vi "ProdaNG.CreateProductComponent.vi"(4 "component serialNo":string, 6 "component wabcoNo":string, 8 "error in (no error)":errorcluster, 9 "product serialNo":string, 10 "product wabcoNo":string, 11 "dbHandle":i32) -> (0 "error out":errorcluster, 3 "dbHandle out":i32)   [LabVIEW 2016]
doc: "This function returns a product structure for a product, which is identified by a part and a serial number.\nImportant information: The field 'individual' was taken over from the field 'allgemein' of the legacy data directly. Because of this most products have the value 0 further on and only a few the value 1. \nParameter:\nhandle is an Integer, which is returned by the function Login() at the creation of a new connection.\nwabcoPartId is the Id of the part.\nserialNumber is the serial number of the product for the part above.\nproduct is a pointer on a product structure, which is filled if the returncode is 0. The structure must be defined in the calling program.\n\nReturncodes:\n0 No error\n< 0 ORACLE Error code\n6 (ERROR_INVALID_HANDLE) in case of an invalid handle\n1403 Record does not exist"
uses:
  Controls/ProdaNG.ProductComponent.ctl
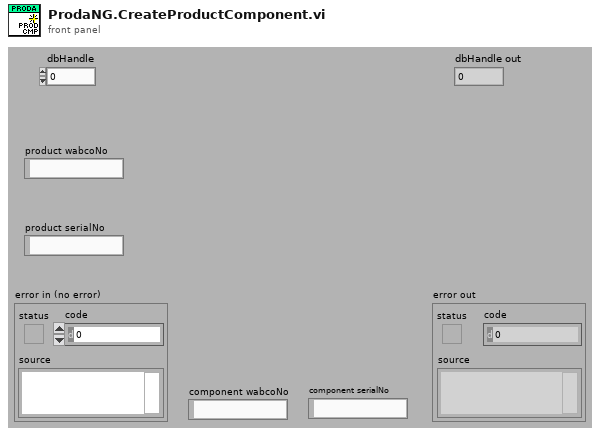
[diagram p1: front panel]
types:
  T1 = typedef "ProdaNG.ProductComponent.ctl" = cluster{"product_wabcoNumber":string, "product_serialNumber":string, "component_wabcoNumber":string, "component_serialNumber":string, "pressStepResultId":string, "qty":i32, "level":i32}
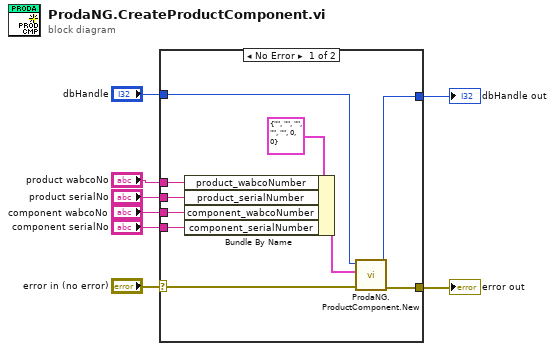
[diagram p0: block diagram]
diagram:
  n1 = case shown="No Error" "error in (no error)" {
    selector: "error in (no error)" -> [w18 w20]
    tunnel: [w17 w20] -> w7
    tunnel: "dbHandle" -> [w16 w19]
    tunnel: [w13 w19] -> w5
    tunnel: "component serialNo" -> [w12 _]
    tunnel: "product serialNo" -> [w10 _]
    tunnel: "component wabcoNo" -> [w9 _]
    tunnel: "product wabcoNo" -> [w11 _]
    frame No Error {
      n2 = Bundle By Name(cluster=T1 {"product_wabcoNumber"="", "product_serialNumber"="", "component_wabcoNumber"="", "component_serialNumber"="", "pressStepResultId"="", "qty"=0, "level"=0} ("Product Component"), "product_wabcoNumber"=w11, "product_serialNumber"=w10, "component_wabcoNumber"=w9, "component_serialNumber"=w12) -> (w15:T1)
      n3 = call "ProdaNG.ProductComponent.New.vi"("error in (no error)"=w18, "Product Component"=w15, "dbHandle"=w16) -> ("error out"=w17:errorcluster, "dbHandle"=w13:i32)  [unwired: 7 in]
    }
    frame Error {
    }
  }
  "error out" <- w7
  "dbHandle out" <- w5
